vi "stopAutomatedTest.vi"(8 "error in (no error)":errorcluster, 10 "model":refnum<class "Model.lvclass">, 11 "AutomatedMotionState in":refnum<class "AutomatedMotionState.lvclass">) -> (0 "error out":errorcluster, 2 "model 2":refnum<class "Model.lvclass">, 3 "AutomatedMotionState out":refnum<class "AutomatedMotionState.lvclass">)   [LabVIEW 2013, in "AutomatedMotionState.lvclass"]
uses:
  AutomatedMotionState.lvclass
  Model/Model/Model.lvclass
  Typedefs/StateSelector.ctl
  Typedefs/M2AADTTypedefs.lvlib
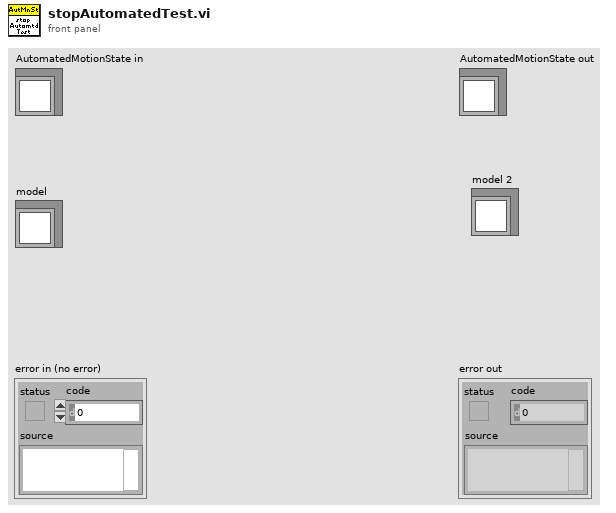
[diagram p1: front panel]
types:
  T1 = typedef "M2AADTTypedefs.lvlib/StateSelector.ctl" = enum16{"EndingCycleState", "FaultState", "InteractiveMotionState", "MovingToNewForceState", "OffState", "PausingState", "StandbyState", "StoppedState"}
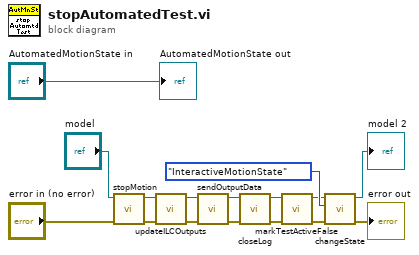
[diagram p0: block diagram]
diagram:
  n1 = call "stopMotion.vi"("error in (no error)"="error in (no error)", "Model in"="model") -> ("error out"=w4:errorcluster, "Model out"=w6:refnum<class "Model.lvclass">)  [unwired: 8 in]
  n2 = call "updateILCOutputs.vi"("error in (no error)"=w4, "Model in"=w6) -> ("error out"=w3:errorcluster, "Model out"=w5:refnum<class "Model.lvclass">)  [unwired: 8 in]
  n3 = call "sendOutputData.vi"("error in (no error)"=w3, "Model in"=w5) -> ("error out"=w1:errorcluster, "Model out"=w2:refnum<class "Model.lvclass">)  [unwired: 8 in]
  n4 = call "closeLog.vi"("error in (no error)"=w1, "Model in"=w2) -> ("error out"=w7:errorcluster, "Model out"=w8:refnum<class "Model.lvclass">)  [unwired: 8 in]
  n5 = call "markTestActiveFalse.vi"("error in (no error)"=w7, "Model in"=w8) -> ("error out"=w9:errorcluster, "Model out"=w10:refnum<class "Model.lvclass">)  [unwired: 8 in]
  n6 = call "changeState.vi"("error in (no error)"=w9, "State:"=StateSelector."InteractiveMotionState", "Model in"=w10) -> ("error out"=→"error out":errorcluster, "Model out"=→"model 2":refnum<class "Model.lvclass">)  [unwired: 7 in]
  "AutomatedMotionState out" <- "AutomatedMotionState in"
